vi "Write Headers_.vi"(8 "error in (no error)":errorcluster, 10 "Headers?":bool, 11 "CSV in":refnum<class "CSV.lvclass">) -> (0 "error out":errorcluster, 3 "CSV out":refnum<class "CSV.lvclass">)   [LabVIEW 2019, in "ManejoArchivos.lvlib" / "CSV.lvclass"]
uses:
  CSV.lvclass
  CSV.lvclass/CSV.ctl
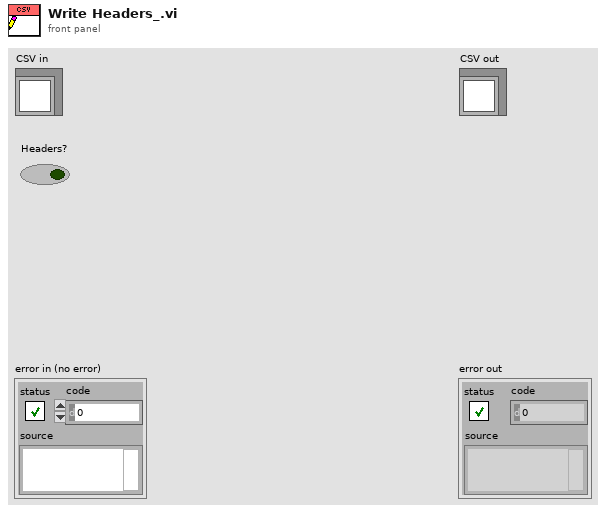
[diagram p1: front panel]
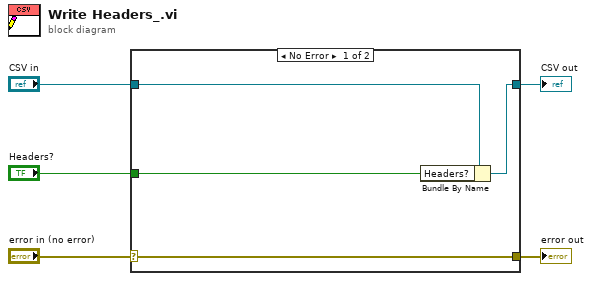
[diagram p0: block diagram]
diagram:
  n1 = case shown="No Error" "error in (no error)" {
    selector: "error in (no error)" -> [w9 w10]
    tunnel: [w9 w10] -> w4
    tunnel: [w7 w11] -> w2
    tunnel: "CSV in" -> [w8 w11]
    tunnel: "Headers?" -> [w6 _]
    frame No Error {
      n2 = Bundle By Name(cluster=w8, "Headers?"=w6) -> (w7:refnum<class "CSV.lvclass">)
    }
    frame Error {
    }
  }
  "error out" <- w4
  "CSV out" <- w2
